vi "Uart test.vi"() -> ()   [LabVIEW 2018]
uses:
  <vilib>/myRIO/Instrument Drivers/Onboard IO/UART/typedef/VISA Configuration.ctl
  <vilib>/myRIO/Common/Instrument Driver Framework/myRIO v1.0/UART/vis/myRIO v1.0 Close UART.vi
  <vilib>/Instr/_visa.llb/VISA Configure Serial Port (Instr).vi
  <vilib>/myRIO/Common/Instrument Driver Framework/Utilities/vis/FPGA Ref Manager.vi
  <vilib>/myRIO/Common/Instrument Driver Framework/myRIO v1.0/myRIO v1.0 Reset FPGA.vi
  <vilib>/myRIO/Common/Instrument Driver Framework/myRIO v1.0/IRQ/vis/myRIO v1.0 IRQ Info FGV.vi
  <vilib>/myRIO/Common/Instrument Driver Framework/myRIO v1.0/IRQ/vis/myRIO v1.0 Timer IRQ Info FGV.vi
  <vilib>/myRIO/Common/Instrument Driver Framework/myRIO v1.0/IRQ/vis/myRIO v1.0 ISR Agent.vi
  <vilib>/myRIO/Express VI/Onboard IO/UART/UART Express VI.xnode
  <vilib>/myRIO/Instrument Drivers/Utilities/Utilities.lvlib
  <vilib>/myRIO/Instrument Drivers/Onboard IO/UART/UART.lvlib
panel:
  out "Mean Lattitude":dbl
  out "Mean Longitude":dbl
  in  "Antal Means":i32=10
  in  "Frekvens":i16=10
  out "Data Array":string[](array[string])
  out "substring 2":string
  out "substring":string
  out "Lattitude":dbl
  out "Longitude":dbl
  out "error out":errorcluster
  in  "stop":bool
  out "Characters Read":string
  # "Aktuel: 10.216"
  # "Aktuel: 56.158"
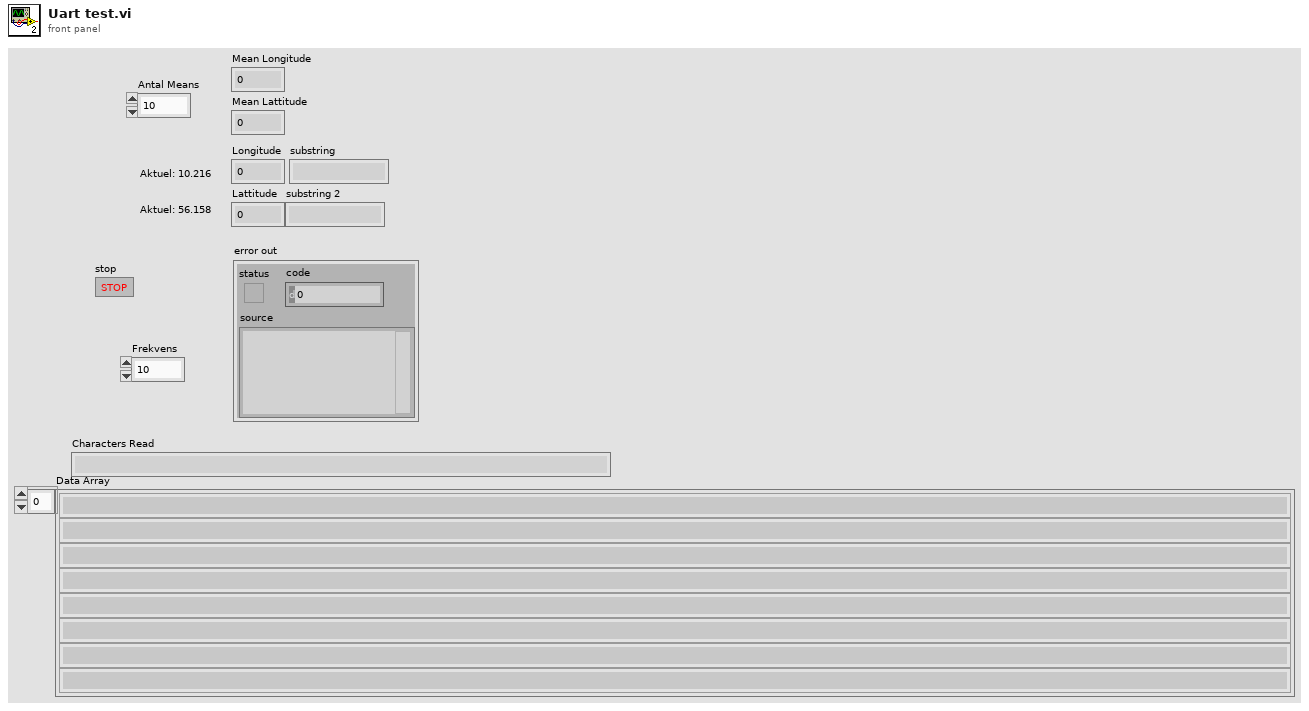
[diagram p1: front panel]
types:
  T1 = typedef "UART.lvlib/VISA Configuration.ctl" = cluster{"baud rate (9600)":u32, "data bits (8)":u16, "parity (0:none)":enum16{"None", "Odd", "Even", "Mark", "Space"}, "stop bits (10: 1 bit)":u16, "flow control (0:none)":u16, "termination char\n(0xA = '\\n' = LF) ":u8, "Enable Termination\nChar (T)":bool, "timeout (10sec)":u32}
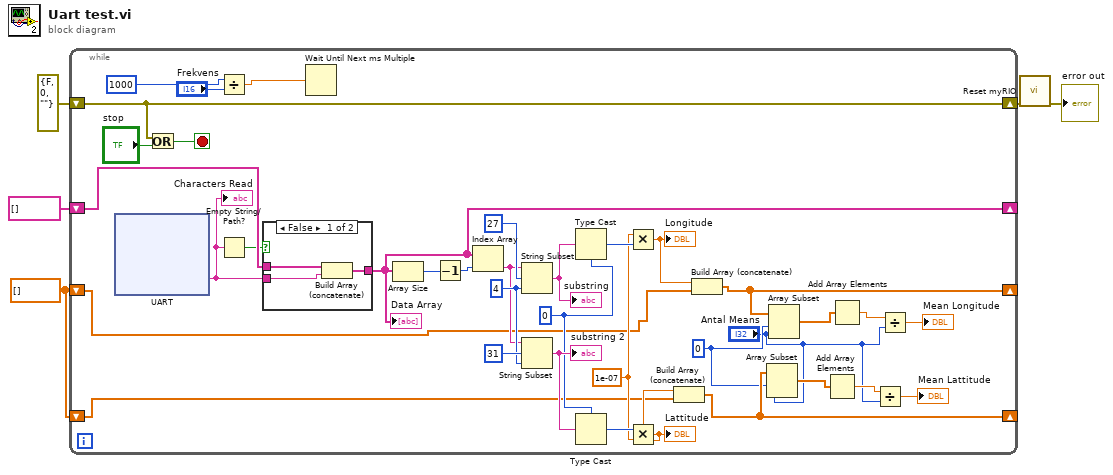
[diagram p0: block diagram]
diagram:
  w1 = dbl[] []
  n1 = while {
    shift-right: [w39] -> w3
    shift-left: errorcluster {"status"=FALSE, "code"=0, "source"=""} ("error out") -> [w39]
    shift-right: [w26] -> _
    shift-left: string[] [] -> [w38]
    shift-right: [w15] -> _
    shift-left: w1 -> [w16]
    shift-right: [w14] -> _
    shift-left: w1 -> [w17]
    stop <- w40 stop-if-true
    w13 = 0
    w27 = 1e-07
    w30 = 0
    w33 = 4 ("length (rest)")
    n2 = xnode "UART"() -> ("Characters Read"=w35:string)  [unwired: 1 in, 1 out]
    "Characters Read" <- w35
    n3 = Or(x=w39, y="stop") -> (x .or. y?=w40:bool)
    n4 = Divide(x=i16 1000 ("milliseconds to wait"), y="Frekvens") -> (x/y=w20:dbl)
    n5 = Empty String/Path?(string/path=w35) -> (empty?=w37:bool)
    n6 = case shown="False" w37 {
      tunnel: w38 -> [w44 w45]
      tunnel: [w43 w45] -> w26
      tunnel: w35 -> [w42 _]
      frame False {
        n7 = Build Array (concatenate)(w44, w42) -> (w43:string[])
      }
      frame True {
      }
    }
    "Data Array" <- w26
    n8 = Wait Until Next ms Multiple(millisecond multiple=w20) -> ()  [unwired: 1 out]
    n9 = Array Size(array=w26) -> (size(s)=w24:i32)
    n10 = Decrement(x=w24) -> (x-1=w23:i32)
    n11 = Index Array(array=w26, index=w23) -> (element=w25:string)
    n12 = String Subset(string=w25, offset (0)=27, length (rest)=w33) -> (substring=w32:string)
    "substring" <- w32
    n13 = String Subset(string=w25, offset (0)=31, length (rest)=w33) -> (substring=w31:string)
    "substring 2" <- w31
    n14 = Type Cast(type=w30, x=w32) -> (*(type *) &x=w28:i32)
    n15 = Type Cast(type=w30, x=w31) -> (*(type *) &x=w29:i32)
    n16 = Multiply(x=w27, y=w28) -> (x*y=w19:dbl)
    "Longitude" <- w19
    n17 = Multiply(x=w29, y=w27) -> (x*y=w18:dbl)
    "Lattitude" <- w18
    n18 = Build Array (concatenate)(w18, w17) -> (w14:dbl[])
    n19 = Build Array (concatenate)(w19, w16) -> (w15:dbl[])
    n20 = Array Subset(array=w14, index=w13, length="Antal Means") -> (w10:dbl[])
    n21 = Array Subset(array=w15, index=w13, length="Antal Means") -> (w9:dbl[])
    n22 = Add Array Elements(numeric array=w10) -> (sum=w11:dbl)
    n23 = Add Array Elements(numeric array=w9) -> (sum=w12:dbl)
    n24 = Divide(x=w11, y="Antal Means") -> (x/y=→"Mean Lattitude":dbl)
    n25 = Divide(x=w12, y="Antal Means") -> (x/y=→"Mean Longitude":dbl)
  }
  n26 = call <vilib>:"Reset myRIO.vi"("error in (no error)"=w3) -> ("error out"=→"error out":errorcluster)  [unwired: 10 in]
